vi "CRYStep Pic Setup Replace .vi"(6 "sOption Etc":string, 7 "sAction":string, 8 "nData":i32, 9 "sStepName":string, 11 "sOption":string) -> (0 "nData_Out":i32)   [LabVIEW 2013]
uses:
  CRYProject Editor Global.vi
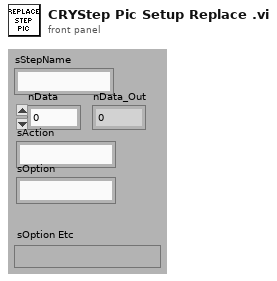
[diagram p1: front panel]
types:
  T1 = typedef "CRYStep.ctl" = cluster{"No.VI":i32, "Category":string, "StepName":string, "Seq setup flattened":string, "Comment":string, "Steps config.":bool[], "Jump config":i32[], "Start":dbl, "Increment":dbl, "Name":string, "Unit":string, "Y data":u16, "Y prefix":string, "Y dB ref":dbl, "Y unit":string, "Repeat State Array":cluster{"Start":dbl, "Increment":dbl, "Count":i32, "Num":i32}[]}
  T2 = cluster{"EventName":string, "Arg1":string, "Numeric":u16, "Numeric 2":u16, "AddSteps ":refnum<vi>, "Arg1 2":string, "Arg1 3":string, "Boolean":bool}
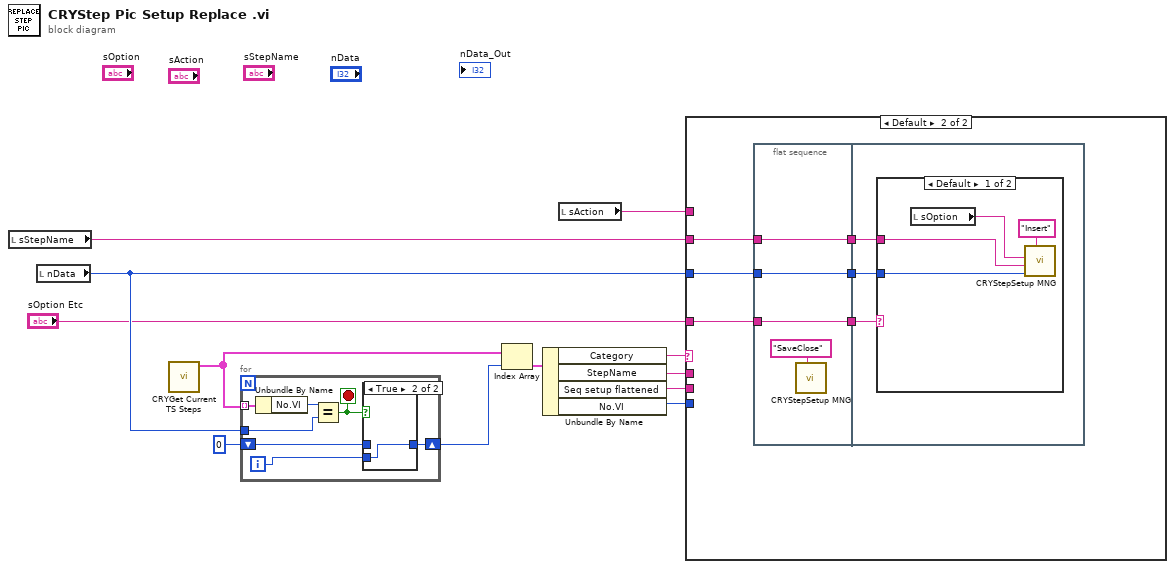
[diagram p0: block diagram]
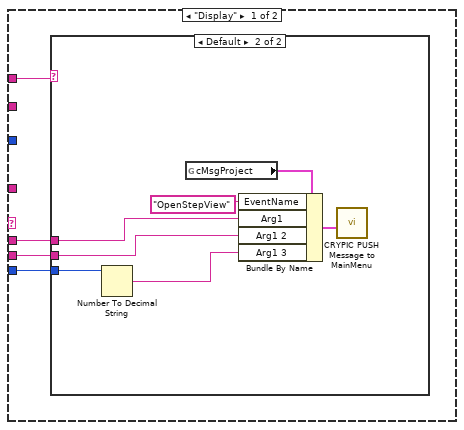
[diagram p2: hidden frame]
diagram:
  n1 = local read "sStepName"() -> (w7:string)
  n2 = local read "nData"() -> (w6:i32)
  n3 = call "CRYGet Current TS Steps.vi"() -> ("Steps"=w11:T1[])  [unwired: 1 in, 10 out]
  n4 = for {
    tunnel: w11 -> [w19] mode=indexing
    tunnel: w6 -> [w17]
    shift-right: [w14] -> w10
    shift-left: 0 -> [w16]
    i -> [w13]
    stop <- w15 stop-if-true
    n5 = Unbundle By Name(w19) -> ("No.VI"=w18:i32)
    n6 = Equal?(x=w18, y=w17) -> (x = y?=w15:bool)
    n7 = case shown="True" w15 {
      tunnel: w16 -> [w20 _]
      tunnel: [w20 w21] -> w14
      tunnel: w13 -> [_ w21]
      frame False {
      }
      frame True {
      }
    }
  }
  n8 = Index Array(array=w11, index=w10) -> (element=w9:T1)
  n9 = Unbundle By Name(w9) -> ("Category"=w8:string, "StepName"=w5:string, "Seq setup flattened"=w4:string, "No.VI"=w2:i32)
  n10 = local read "sAction"() -> (w3:string)
  n11 = case shown="Default" w8 {
    tunnel: w7 -> [_ w38]
    tunnel: w6 -> [_ w37]
    tunnel: w5 -> [w25 _]
    tunnel: w4 -> [w24 _]
    tunnel: w3 -> [w23 _]
    tunnel: w2 -> [w22 _]
    tunnel: "sOption Etc" -> [_ w34]
    frame "Display" {
      n12 = case shown="Default" w23 {
        tunnel: w25 -> [_ w32]
        tunnel: w24 -> [_ w31]
        tunnel: w22 -> [_ w30]
        frame "SkipDisplay" {
        }
        frame Default {
          n13 = Number To Decimal String(number=w30) -> (decimal integer string=w27:string)  [unwired: 1 in]
          n14 = global read "CRYProject Editor Global.vi" "cMsgProject"() -> (w29:T2)
          n15 = Bundle By Name(cluster=w29, "EventName"="OpenStepView", "Arg1"=w32, "Arg1 2"=w31, "Arg1 3"=w27) -> (w26:T2)
          n16 = call "CRYPIC PUSH Message to MainMenu.vi"("cMsgProject"=w26) -> ()  [unwired: 11 in]
        }
      }
    }
    frame Default {
      n17 = flat-sequence {
        tunnel: w38 -> [w41]
        tunnel: w37 -> [w40]
        tunnel: [w41] -> w36
        tunnel: [w40] -> w35
        tunnel: w34 -> [w39]
        tunnel: [w39] -> w33
        tunnel: w36 -> [w45]
        tunnel: w35 -> [w44]
        tunnel: w33 -> [w43]
        frame #0 {
          n18 = call "CRYStepSetup MNG.vi"("sAction"="SaveClose") -> ()  [unwired: 9 in, 2 out]
        }
        frame #1 {
          n19 = case shown="Default" w43 {
            tunnel: w45 -> [w49 _]
            tunnel: w44 -> [w48 _]
            frame Default {
              n20 = local read "sOption"() -> (w47:string)
              n21 = call "CRYStepSetup MNG.vi"("sAction"="Insert", "nData"=w48, "sStepName"=w49, "sOption"=w47) -> ()  [unwired: 6 in, 2 out]
            }
            frame "StepRemove" {
            }
          }
        }
      }
    }
  }
